vi "XY Graph Invert Plots Selection Event.vi"(8 "Error In":errorcluster, 11 "XYGraph Ref":T1) -> (0 "Error Out":errorcluster, 1 "Message":string, 3 "XYGraph Ref":T1, 5 "Graph Name":string)   [LabVIEW 2019, in "XY Graph Add-Ons.lvlib"]
uses:
  XY Graph Add-Ons.lvlib
  XY Graph Refnum.ctl
  <vilib>/Utility/High Resolution Relative Seconds.vi
panel:
  out "CPU (s)":dbl
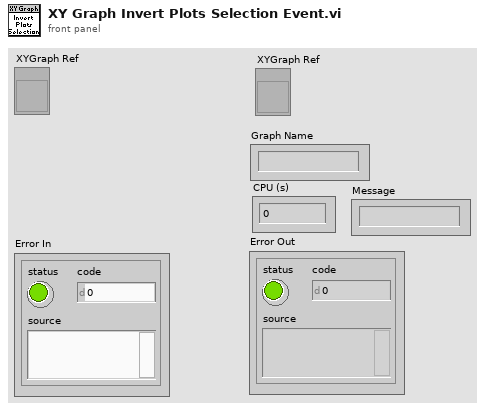
[diagram p1: front panel]
types:
  T1 = typedef "XY Graph Add-Ons.lvlib/XY Graph Refnum.ctl" = refnum<vi>
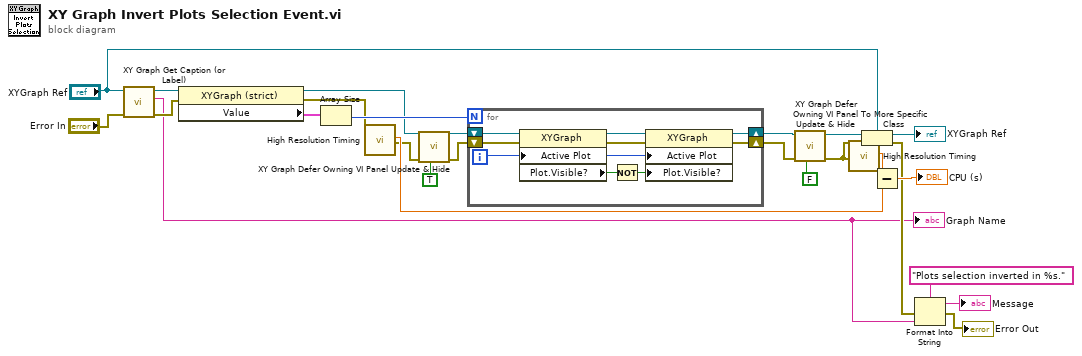
[diagram p0: block diagram]
diagram:
  n1 = call "XY Graph Get Caption (or Label).vi"("error in (no error)"="Error In", "XYGraph in"="XYGraph Ref") -> ("error out"=w2:errorcluster, "Caption (or Label) Text"=w1:string, "XYGraph out"=w3:T1)  [unwired: 7 in]
  "Graph Name" <- w1
  n2 = property class="XYGraph (strict)"(reference=w3, error in=w2) -> (reference out=w24:T1, error out=w23:errorcluster, "Value"=w26:cluster{"X Array":dbl[], "Y Array":dbl[]}[])
  n3 = Array Size(array=w26) -> (size(s)=w25:i32)
  n4 = call "High Resolution Timing.vi"("Error In"=w23) -> ("elapsed (relative) seconds"=w21:dbl, "Error Out"=w18:errorcluster)  [unwired: 16 in, 1 out]
  n5 = call "XY Graph Defer Owning VI Panel Update & Hide.vi"("Defer Owning Panel Update"=TRUE ("Hide (F)/Show (T) Graph"), "error in (no error)"=w18, "XY Graph Refnum in"=w24) -> ("error out"=w17:errorcluster, "XY Graph Refnum out"=w19:refnum<vi>)  [unwired: 7 in]
  n6 = for {
    N: w25 -> [_]
    shift-right: [w31] -> w16
    shift-left: w19 -> [w35]
    shift-right: [w30] -> w15
    shift-left: w17 -> [w34]
    i -> [w29]
    n7 = property class="XYGraph"(reference=w35, error in=w34, "Active Plot"=w29) -> (reference out=w33:refnum<vi>, error out=w32:errorcluster, "Plot.Visible?"=w28:bool)
    n8 = Not(x=w28) -> (.not. x?=w27:bool)
    n9 = property class="XYGraph"(reference=w33, error in=w32, "Active Plot"=w29, "Plot.Visible?"=w27) -> (reference out=w31:refnum<vi>, error out=w30:errorcluster)
  }
  n10 = call "XY Graph Defer Owning VI Panel Update & Hide.vi"("Defer Owning Panel Update"=FALSE ("Hide (F)/Show (T) Graph"), "error in (no error)"=w15, "XY Graph Refnum in"=w16) -> ("error out"=w12:errorcluster, "XY Graph Refnum out"=w14:refnum<vi>)  [unwired: 7 in]
  n11 = call "High Resolution Timing.vi"("Error In"=w12) -> ("elapsed (relative) seconds"=w22:dbl)  [unwired: 16 in, 2 out]
  n12 = To More Specific Class(target class="XYGraph Ref", reference=w14, error in=w12) -> (specific class reference=→"XYGraph Ref":T1, error out=w9:errorcluster)
  n13 = Subtract(x=w22, y=w21) -> (x-y=→"CPU (s)":dbl)
  n14 = Format Into String(format string="Plots selection inverted in %s.", error in=w9, w1) -> (resulting string=→"Message":string, error out=→"Error Out":errorcluster)  [unwired: 1 in]
